vi "Read config COM.vi"(8 "Path":string, 11 "Settings WT1600 ing":T1={"data bits"=8, "parity"=0, "stop bits"=10, "flow control"=0, "baud rate"=8, "COM"=""} {"baud rate" min=5 max=8 step=1; "flow control" items=["None"=0, "XON/XOFF"=1, "RTS/CTS"=2, "DTR/DSR"=4]; "stop bits" items=["1.0"=10, "1.5"=15, "2.0"=20]; "parity" items=["None", "Odd", "Even", "Mark", "Space"]; "data bits" min=5 max=8 step=1}) -> (3 "Settings WT1600 out":T1={"data bits"=8, "parity"=0, "stop bits"=10, "flow control"=0, "baud rate"=8, "COM"=""} {"baud rate" min=5 max=8 step=1; "flow control" items=["None"=0, "XON/XOFF"=1, "RTS/CTS"=2, "DTR/DSR"=4]; "stop bits" items=["1.0"=10, "1.5"=15, "2.0"=20]; "parity" items=["None", "Odd", "Even", "Mark", "Space"]; "data bits" min=5 max=8 step=1})   [LabVIEW 2019]
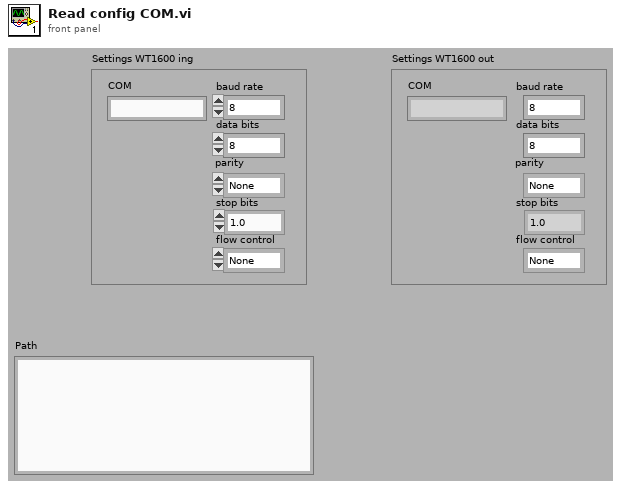
[diagram p1: front panel]
types:
  T1 = cluster{"data bits":u16, "parity":u16, "stop bits":u16, "flow control":u16, "baud rate":u16, "COM":string}
  T2 = enum16{"open", "replace", "create", "open or create", "replace or create", "replace or create with confirmation"}
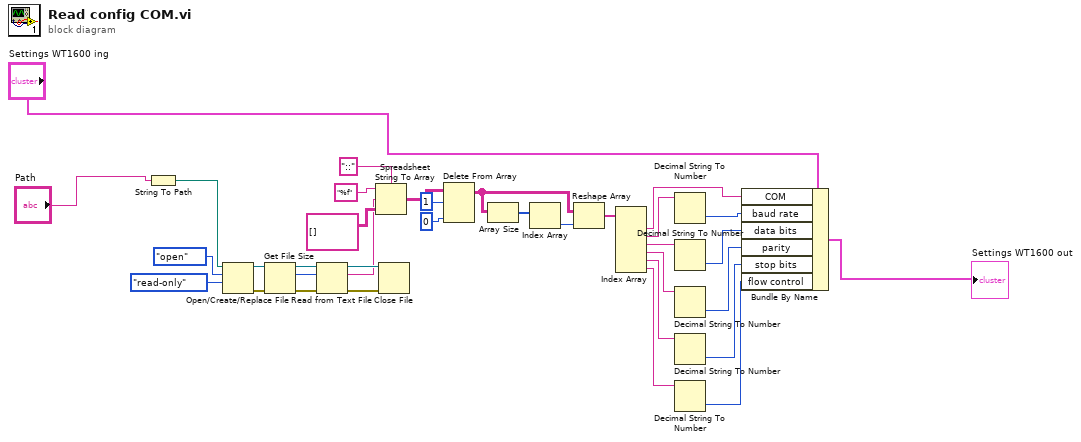
[diagram p0: block diagram]
diagram:
  n1 = String To Path(string="Path") -> (path=w20:path)
  n2 = Open/Create/Replace File(file path (use dialog)=w20, operation (0:open)=T2."open", access (0:read/write)=enum16{"read/write", "read-only", "write-only"}."read-only") -> (refnum out=w25:refnum<file>, error out=w26:errorcluster)  [unwired: 1 in, 3 out]
  n3 = Get File Size(file=w25, error in=w26) -> (refnum out=w24:refnum<file>, size (in bytes)=w23:i64, 0:w22:errorcluster)
  n4 = Read from Text File(file (use dialog)=w24, count=w23, error in=w22) -> (refnum out=w30:refnum<file>, text=w28:string, error out=w29:errorcluster)  [unwired: 2 out]
  n5 = Spreadsheet String To Array(delimiter (Tab)="::", format string="%f", spreadsheet string=w28, array type (2D Dbl)=string[][] [] ("Array")) -> (array=w33:string[][])
  n6 = Close File(refnum=w30, error in=w29) -> ()  [unwired: 2 out]
  n7 = Delete From Array(array=w33, length=1, index (col)=0 ("disabled index (col)")) -> (array with subset deleted=w18:string[][])  [unwired: 1 in, 1 out]
  n8 = Array Size(array=w18) -> (size(s)=w17:i32[])
  n9 = Index Array(array=w17) -> (element=w16:i32)  [unwired: 1 in]
  n10 = Reshape Array(w18, w16) -> (w15:string[])
  n11 = Index Array(array=w15) -> (element #1=w9:string, element #2=w8:string, element #3=w7:string, element #4=w6:string, element #5=w5:string, element #6=w4:string)  [unwired: 6 in]
  n12 = Decimal String To Number(string=w8) -> (number=w14:i32)  [unwired: 3 out]
  n13 = Decimal String To Number(string=w7) -> (number=w13:i32)  [unwired: 3 out]
  n14 = Decimal String To Number(string=w6) -> (number=w12:i32)  [unwired: 3 out]
  n15 = Decimal String To Number(string=w5) -> (number=w11:i32)  [unwired: 3 out]
  n16 = Decimal String To Number(string=w4) -> (number=w10:i32)  [unwired: 3 out]
  n17 = Bundle By Name(cluster="Settings WT1600 ing", "COM"=w9, "baud rate"=w14, "data bits"=w13, "parity"=w12, "stop bits"=w11, "flow control"=w10) -> (→"Settings WT1600 out":T1)
